vi "生成DNS数据.vi"(11 "字符串":string) -> (3 "手机号码内容":u8[](array[numeric]) format="%x")   [LabVIEW 2015]
panel:
  out "大小":i32
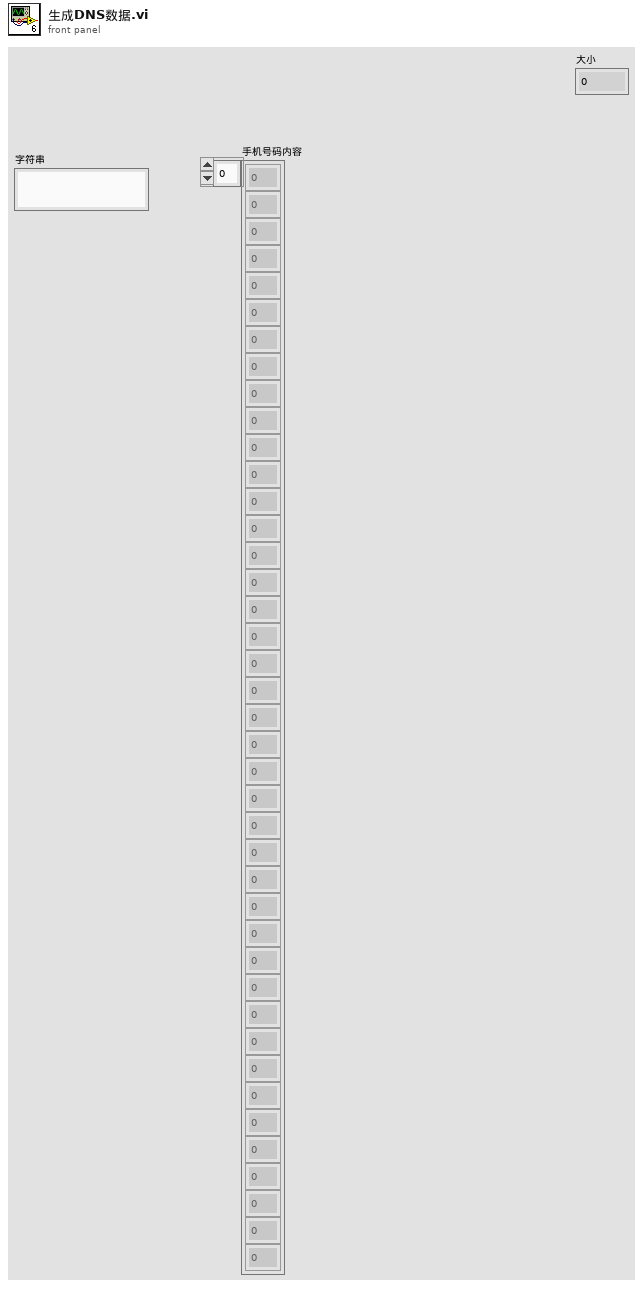
[diagram p1: front panel]
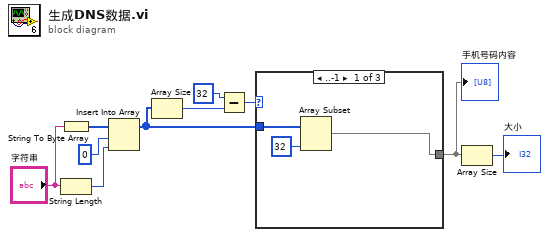
[diagram p0: block diagram]
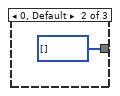
[diagram p2: hidden frame]
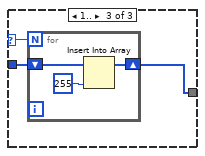
[diagram p3: hidden frame]
diagram:
  n1 = String To Byte Array(string="字符串") -> (unsigned byte array=w8:u8[])
  n2 = String Length(string="字符串") -> (length=w6:i32)
  n3 = Insert Into Array(array=w8, index=0 ("索引"), new element=w6) -> (w2:u8[])
  n4 = Array Size(array=w2) -> (size(s)=w1:i32)
  n5 = Subtract(x=32 ("y"), y=w1) -> (x-y=w5:i32)
  n6 = case shown="..-1" w5 {
    selector: w5 -> [_ _ w17]
    tunnel: w2 -> [w13 _ w16]
    tunnel: [w11 u8[] [] ("unsigned byte array") w15] -> w4
    frame ..-1 {
      n7 = Array Subset(array=w13, length=32 ("长度")) -> (w11:u8[])  [unwired: 1 in]
    }
    frame 0, Default {
    }
    frame 1.. {
      n8 = for {
        N: w17 -> [_]
        shift-right: [w20] -> w15
        shift-left: w16 -> [w19]
        n9 = Insert Into Array(array=w19, new element=u8 255 ("新元素/子数组")) -> (w20:u8[])  [unwired: 1 in]
      }
    }
  }
  "手机号码内容" <- w4
  n10 = Array Size(array=w4) -> (size(s)=→"大小":i32)
